vi "Dbl precision.vi"(10 "precision (6)":i16, 11 "Numeric in":dbl) -> (3 "Numeric out":dbl)   [LabVIEW 2019]
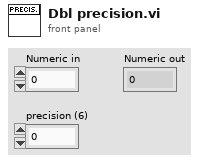
[diagram p1: front panel]
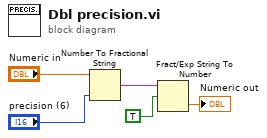
[diagram p0: block diagram]
diagram:
  n1 = Number To Fractional String(number="Numeric in", precision (6)="precision (6)") -> (F-format string=w3:string)  [unwired: 2 in]
  n2 = Fract/Exp String To Number(use system decimal point (T)=TRUE, string=w3) -> (number=→"Numeric out":dbl)  [unwired: 2 in, 1 out]
